vi "Format Cell Range to Named Range.vi"(11 "Cell Range":string) -> (3 "Formatted Cell Range":string)   [LabVIEW 2019, in "Open Xml.lvlib"]
uses:
  Open Xml.lvlib
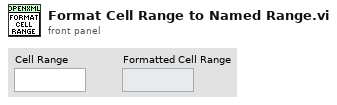
[diagram p1: front panel]
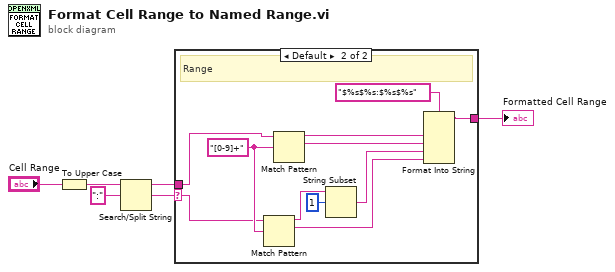
[diagram p0: block diagram]
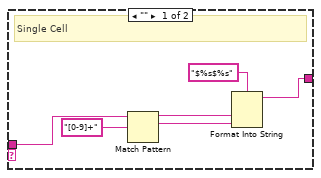
[diagram p2: hidden frame]
diagram:
  n1 = To Upper Case(1:"Cell Range") -> (0:w3:string)
  n2 = Search/Split String(string=w3, search string/char (-)=":") -> (substring before match=w5:string, match + rest of string=w2:string)  [unwired: 1 in, 1 out]
  n3 = case shown="Default" w2 {
    selector: w2 -> [_ w21]
    tunnel: w5 -> [w9 w23]
    tunnel: [w11 w15] -> w1
    frame "" {
      # "Single Cell"
      n4 = Match Pattern(string=w9, regular expression="[0-9]+") -> (before substring=w8:string, match substring=w7:string)  [unwired: 1 in, 2 out]
      n5 = Format Into String(format string="$%s$%s", w8, w7) -> (resulting string=w11:string)  [unwired: 2 in, 1 out]
    }
    frame Default {
      w22 = "[0-9]+" ("regular expression")
      # "Range"
      n6 = Match Pattern(string=w21, regular expression=w22) -> (before substring=w17:string, match substring=w16:string)  [unwired: 1 in, 2 out]
      n7 = Match Pattern(string=w23, regular expression=w22) -> (before substring=w20:string, match substring=w18:string)  [unwired: 1 in, 2 out]
      n8 = String Subset(string=w17, offset (0)=1) -> (substring=w14:string)  [unwired: 1 in]
      n9 = Format Into String(format string="$%s$%s:$%s$%s", w20, w18, w14, w16) -> (resulting string=w15:string)  [unwired: 2 in, 1 out]
    }
  }
  "Formatted Cell Range" <- w1
